vi "H5Tarray_create.vi"(6 "error in (no error)":errorcluster, 7 "Dimensions":u64[](array[numeric]), 8 "HDF5 Base Type Ref":T1) -> (0 "error out":errorcluster, 3 "HDF5 Array Type out":T1)   [LabVIEW 2017]
doc: "Creates an array datatype object."
uses:
  <vilib>/UPVI/lvhdf5/library.llb/HDF5 Ref.ctl
  <vilib>/UPVI/lvhdf5/hdf5.dll
panel:
  # "LVHDF5 Toolkit\nCopyright (c) 2005-2013 by Jason D. Sommerville\nCopyright (c) 2014 by UPVI, LLC.\n\nThis use and distribution of this file is governed by the terms found in \nLICENSE.txt distributed with this toolkit and installed at\n <user.lib>\\_lvhdf5\\LICENSE.txt"
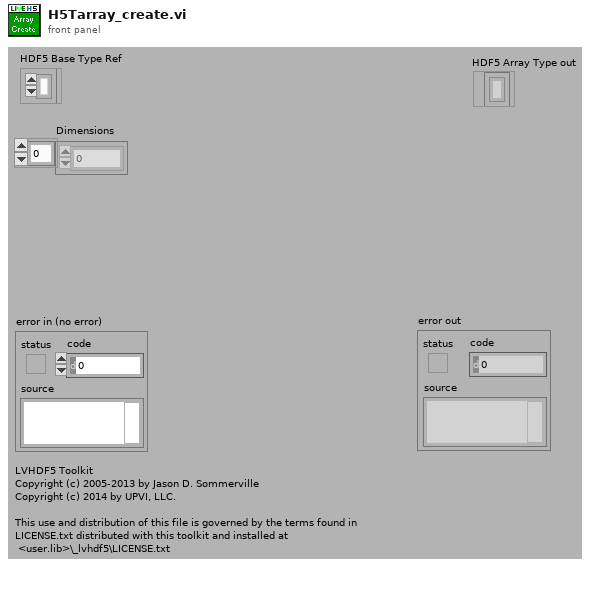
[diagram p1: front panel]
types:
  T1 = typedef "HDF5 Ref.ctl" = refnum<k1>
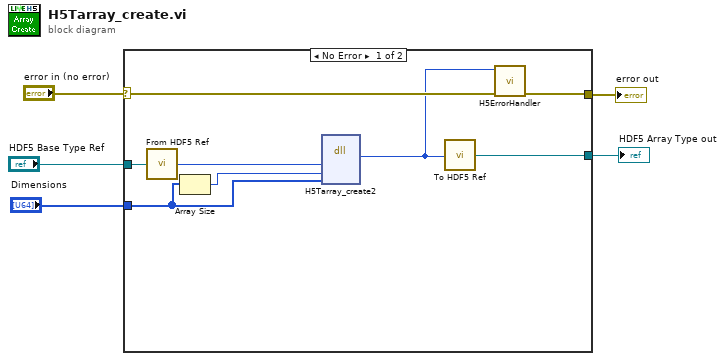
[diagram p0: block diagram]
diagram:
  n1 = case shown="No Error" "error in (no error)" {
    selector: "error in (no error)" -> [w13 w14]
    tunnel: [w12 w14] -> w4
    tunnel: "HDF5 Base Type Ref" -> [w11 _]
    tunnel: [w8 _] -> w2
    tunnel: "Dimensions" -> [w6 _]
    frame No Error {
      n2 = call <vilib>:"From HDF5 Ref.vi"("HDF5 Ref"=w11) -> ("I32"=w10:i32)
      n3 = Array Size(array=w6) -> (size(s)=w7:i32)
      n4 = dll-call lib="C:/Program Files/National Instruments/LabVIEW 2017/vi.lib/UPVI/lvhdf5/hdf5.dll" fn="H5Tarray_create2" label="H5Tarray_create"("base"=w10, "rank"=w7, "dims"=w6) -> ("return type"=w9:i32)  [unwired: 6 in, 2 out]
      n5 = call <vilib>:"To HDF5 Ref.vi"("I32"=w9) -> ("HDF5 Ref"=w8:T1)
      n6 = call <vilib>:"H5ErrorHandler.vi"("error in (no error)"=w13, "herr_t"=w9) -> ("error out"=w12:errorcluster)  [unwired: 3 in, 4 out]
    }
    frame Error {
    }
  }
  "error out" <- w4
  "HDF5 Array Type out" <- w2
